vi "Main.vi"() -> ()   [LabVIEW 2019]
uses:
  Global Variables/global.vi
  Instrument_Setup.vi
  Global Variables/Data_Display_global.vi
panel:
  out "Main Iter. Index":i32
  # "CryoTUM  VTI/JT"
  # "Stop messung\nnach diese\nMessreihe"
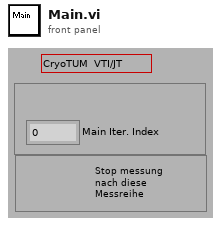
[diagram p1: front panel]
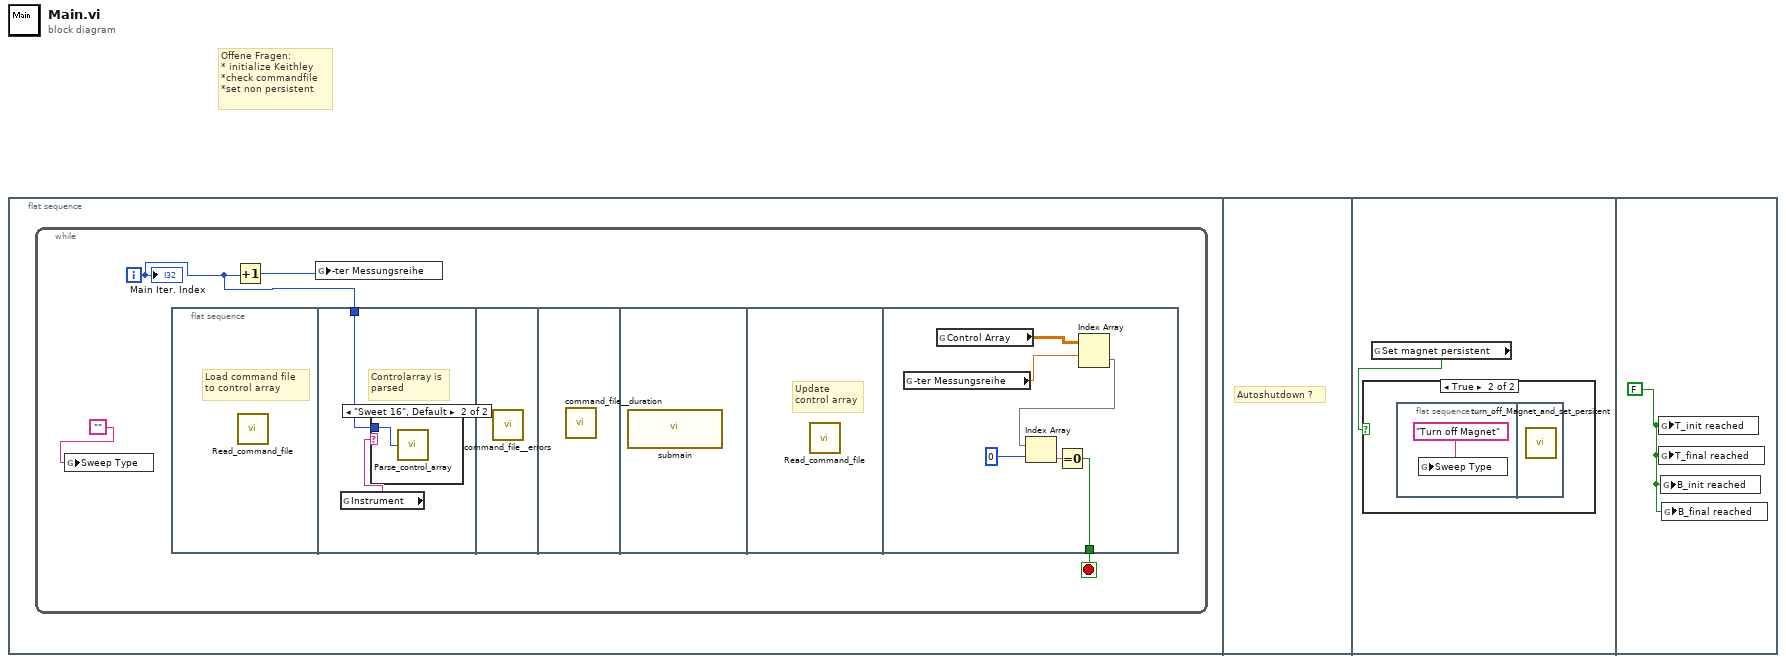
[diagram p0: block diagram]
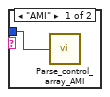
[diagram p2: hidden frame]
diagram:
  # "Offene Fragen:\n* initialize Keithley\n*check commandfile\n*set non persistent"
  n1 = flat-sequence {
    frame #0 {
      n2 = while {
        i -> [w2]
        stop <- w4 stop-if-true
        n3 = global write "global.vi" "Sweep Type"("") -> ()
        n4 = flat-sequence {
          tunnel: w2 -> [w6]
          tunnel: [w9] -> w4
          frame #0 {
            # "Load command file\nto control array"
            n5 = call "Read_command_file.vi"() -> ()  [unwired: 12 in]
          }
          frame #1 {
            # "Controlarray is\nparsed"
            n6 = global read "Instrument_Setup.vi" "Instrument"() -> (w5:string)
            n7 = case shown="\"Sweet 16\", Default" w5 {
              tunnel: w6 -> [w7 w8]
              frame "AMI" {
                n8 = call "Parse_control_array_AMI.vi"("Messreihe"=w7) -> ()  [unwired: 1 in]
              }
              frame "Sweet 16", Default {
                n9 = call "Parse_control_array.vi"("Messreihe"=w8) -> ()  [unwired: 1 in]
              }
            }
          }
          frame #2 {
            n10 = call "command_file__errors.vi"() -> ()  [unwired: 12 in]
          }
          frame #3 {
            n11 = call "command_file__duration.vi"() -> ()  [unwired: 12 in]
          }
          frame #4 {
            n12 = call "submain.vi"() -> ()  [unwired: 4 in]
          }
          frame #5 {
            # "Update\ncontrol array"
            n13 = call "Read_command_file.vi"() -> ()  [unwired: 12 in]
          }
          frame #6 {
            n14 = global read "global.vi" "-ter Messungsreihe"() -> (w14:dbl)
            n15 = global read "global.vi" "Control Array"() -> (w12:dbl[][])
            n16 = Index Array(array=w12, index (row)=w14) -> (element=w13:dbl[])  [unwired: 1 in]
            n17 = Index Array(array=w13, index=0) -> (element=w11:dbl)
            n18 = Equal To 0?(x=w11) -> (x = 0?=w9:bool)
          }
        }
        n19 = Increment(x=w2) -> (x+1=w3:i32)
        n20 = global write "global.vi" "-ter Messungsreihe"(w3) -> ()
        "Main Iter. Index" <- w2
      }
    }
    frame #1 {
      # "Autoshutdown ?"
    }
    frame #2 {
      n21 = global read "Instrument_Setup.vi" "Set magnet persistent"() -> (w15:bool)
      n22 = case shown="True" w15 {
        frame False {
        }
        frame True {
          n23 = flat-sequence {
            frame #0 {
              n24 = global write "global.vi" "Sweep Type"("Turn off Magnet") -> ()
            }
            frame #1 {
              n25 = call "turn_off_Magnet_and_set_persitent.vi"() -> ()  [unwired: 4 in]
            }
          }
        }
      }
    }
    frame #3 {
      w17 = FALSE ("T_init reached")
      n26 = global write "Data_Display_global.vi" "T_init reached"(w17) -> ()
      n27 = global write "Data_Display_global.vi" "T_final reached"(w17) -> ()
      n28 = global write "Data_Display_global.vi" "B_init reached"(w17) -> ()
      n29 = global write "Data_Display_global.vi" "B_final reached"(w17) -> ()
    }
  }
